vi "get_dataConverter.vi"(0 "HGV_PVBase":refnum<class "HGF_PVBase.lvclass">, 5 "error in (no error)":errorcluster) -> (14 "dup HGV_PVBase":refnum<class "HGF_PVBase.lvclass">, 16 "HGF_PVDataConverter":refnum<class "HGF_PVDataConverter.lvclass">, 19 "error out":errorcluster)   [LabVIEW 2014, in "HGF_BaseClasses.lvlib" / "HGF_PVBase.lvclass"]
doc: "Get DataConverter object"
uses:
  HGF_PVBase.lvclass
  HGF_PVDataConverter/HGF_PVDataConverter.lvclass
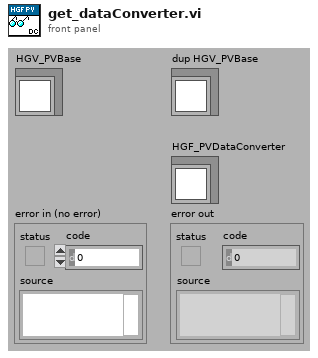
[diagram p1: front panel]
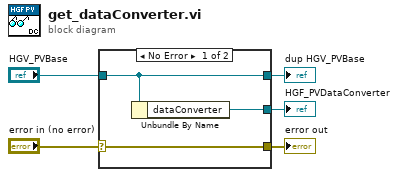
[diagram p0: block diagram]
diagram:
  n1 = case shown="No Error" "error in (no error)" {
    selector: "error in (no error)" -> [w8 w9]
    tunnel: [w8 w9] -> w4
    tunnel: [w7 w10] -> w2
    tunnel: "HGV_PVBase" -> [w7 w10]
    tunnel: [w6 _] -> w1
    frame No Error {
      n2 = Unbundle By Name(w7) -> ("dataConverter"=w6:refnum<class "HGF_PVDataConverter.lvclass">)
    }
    frame Error {
    }
  }
  "error out" <- w4
  "dup HGV_PVBase" <- w2
  "HGF_PVDataConverter" <- w1
